vi "Convierte un hexadecimal a un ip.vi"() -> ()   [LabVIEW 2019]
panel:
  out "concatenated string":string
  out "substring 4":string
  out "number 4":u32
  out "substring 3":string
  out "number 3":u32
  out "substring 2":string
  out "number 2":u32
  out "number":u32
  out "substring":string
  out "hex integer string":string
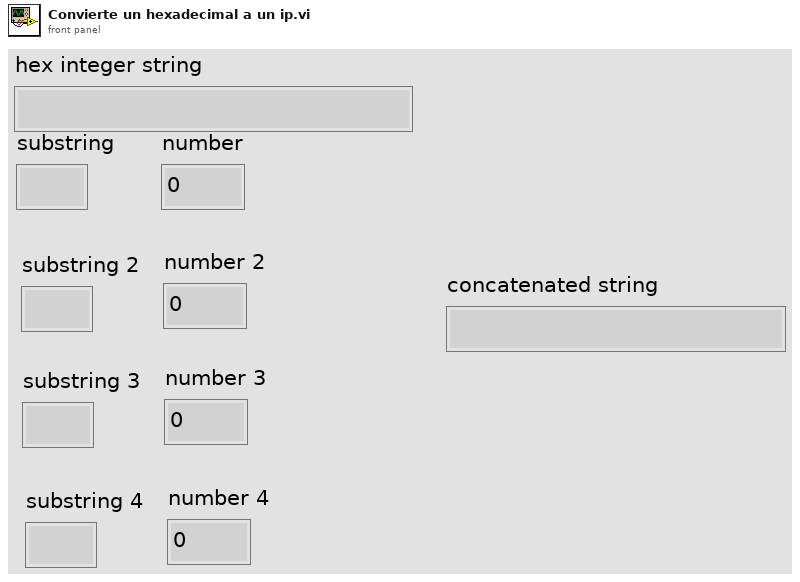
[diagram p1: front panel]
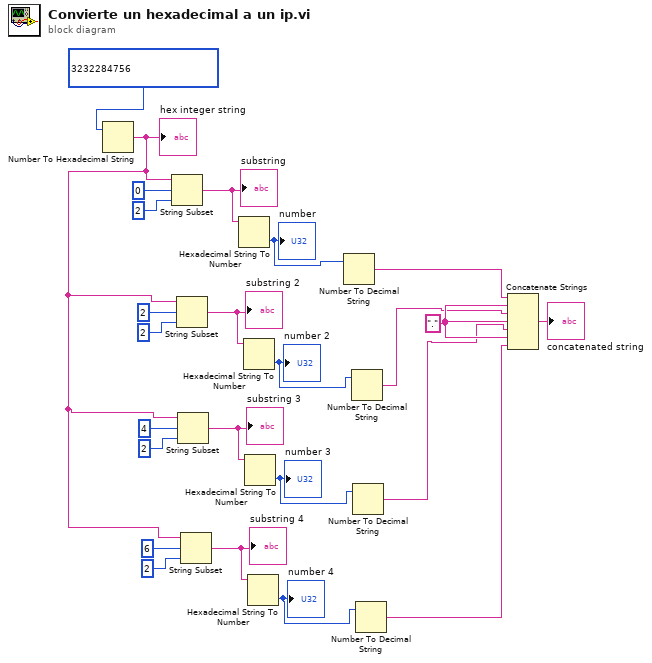
[diagram p0: block diagram]
diagram:
  w10 = "."
  n1 = Number To Hexadecimal String(2:u32 3232284756 ("net address")) -> (0:w11:string)  [unwired: 1 in]
  "hex integer string" <- w11
  n2 = String Subset(string=w11, offset (0)=0, length (rest)=2 ("length (rest)")) -> (substring=w21:string)
  "substring" <- w21
  n3 = String Subset(string=w11, offset (0)=2, length (rest)=2 ("length (rest)")) -> (substring=w20:string)
  "substring 2" <- w20
  n4 = String Subset(string=w11, offset (0)=4, length (rest)=2 ("length (rest)")) -> (substring=w15:string)
  "substring 3" <- w15
  n5 = String Subset(string=w11, offset (0)=6, length (rest)=2 ("length (rest)")) -> (substring=w14:string)
  "substring 4" <- w14
  n6 = Hexadecimal String To Number(string=w21) -> (number=w9:u32)  [unwired: 2 in, 1 out]
  "number" <- w9
  n7 = Hexadecimal String To Number(string=w20) -> (number=w8:u32)  [unwired: 2 in, 1 out]
  "number 2" <- w8
  n8 = Hexadecimal String To Number(string=w15) -> (number=w7:u32)  [unwired: 2 in, 1 out]
  "number 3" <- w7
  n9 = Hexadecimal String To Number(string=w14) -> (number=w6:u32)  [unwired: 2 in, 1 out]
  "number 4" <- w6
  n10 = Number To Decimal String(number=w9) -> (decimal integer string=w5:string)  [unwired: 1 in]
  n11 = Number To Decimal String(number=w8) -> (decimal integer string=w4:string)  [unwired: 1 in]
  n12 = Number To Decimal String(number=w7) -> (decimal integer string=w3:string)  [unwired: 1 in]
  n13 = Number To Decimal String(number=w6) -> (decimal integer string=w2:string)  [unwired: 1 in]
  n14 = Concatenate Strings(w5, w10, w4, w10, w3, w10, w2) -> (→"concatenated string":string)
